vi "Disable Listbox.vi"(8 "error in (no error)":errorcluster, 11 "Listbox Ref":refnum<vi>) -> (0 "error out":errorcluster)   [LabVIEW 2016, in "System Mapping Tool.lvlib"]
uses:
  System Mapping Tool.lvlib
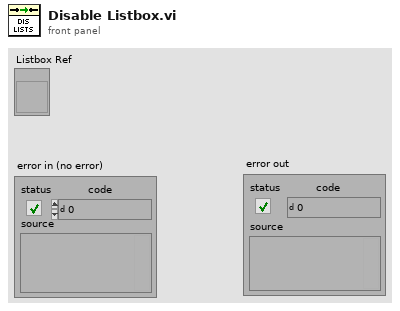
[diagram p1: front panel]
types:
  T1 = enum8{"Enabled", "Disabled", "Disabled and Grayed Out"}
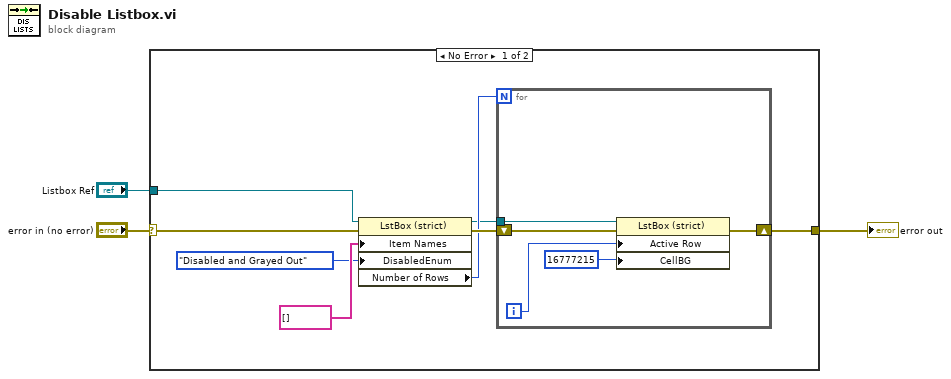
[diagram p0: block diagram]
diagram:
  n1 = case shown="No Error" "error in (no error)" {
    selector: "error in (no error)" -> [w11 w17]
    tunnel: [w4 w17] -> w2
    tunnel: "Listbox Ref" -> [w8 _]
    frame No Error {
      n2 = property class="LstBox (strict)"(reference=w8, error in=w11, "Item Names"=string[] [], "DisabledEnum"=T1."Disabled and Grayed Out" ("Disabled")) -> (reference out=w5:refnum<vi>, error out=w7:errorcluster, "Number of Rows"=w6:u32)
      n3 = for {
        N: w6 -> [_]
        shift-right: [w15] -> w4
        shift-left: w7 -> [w16]
        tunnel: w5 -> [w14]
        i -> [w13]
        n4 = property class="LstBox (strict)"(reference=w14, error in=w16, "Active Row"=w13, "CellBG"=u32 16777215 ("Active Row:Cell Background Color")) -> (error out=w15:errorcluster)  [unwired: 1 out]
      }
    }
    frame Error {
    }
  }
  "error out" <- w2
